vi "sub_SDR_mod.vi"(10 "Array":i16[](array[numeric]), 11 "Modulation Type":enum16{"BPSK", "4-QAM", "16-QAM", "64-QAM"}(ring)) -> (2 "Array out":cdb[](array[numeric]))   [LabVIEW 2012]
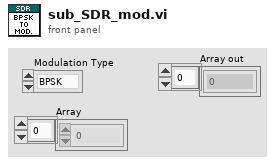
[diagram p1: front panel]
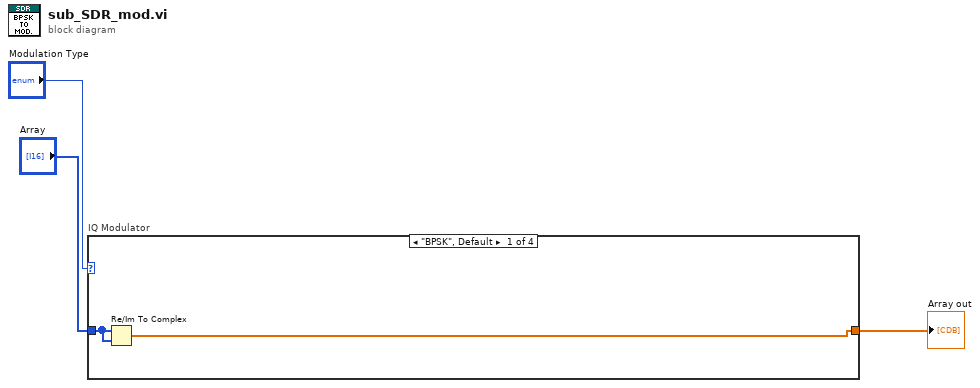
[diagram p0: block diagram]
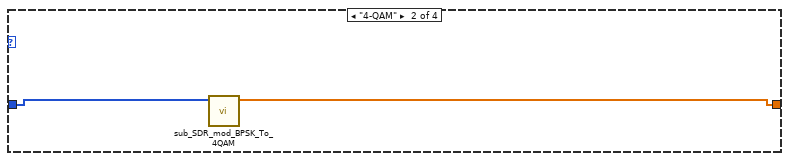
[diagram p2: hidden frame]
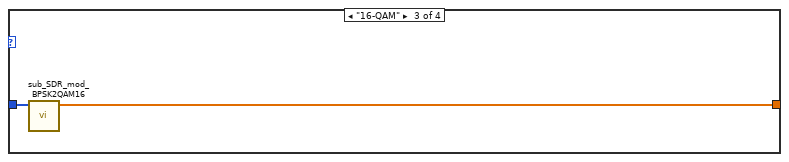
[diagram p3: hidden frame]
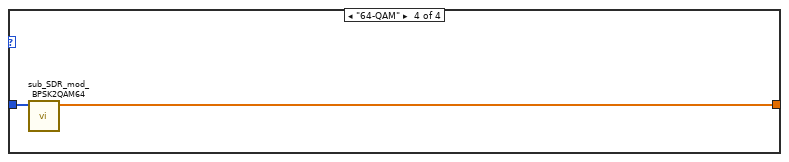
[diagram p4: hidden frame]
diagram:
  n1 = case "IQ Modulator" shown="\"BPSK\", Default" "Modulation Type" {
    tunnel: "Array" -> [w5 w6 w9 w10]
    tunnel: [w4 w7 w8 w11] -> w2
    frame "BPSK", Default {
      # "BPSK Modulator: Convert each input byte array into bolean arrays, sets phase and convert into complex"
      n2 = Re/Im To Complex(1:w5, 2:w5) -> (0:w4:cdb[])
    }
    frame "4-QAM" {
      # "4-QAM Modulator: Convert each byte in 4 integers which are maped in the defined symbols"
      n3 = call "sub_SDR_mod_BPSK_To_4QAM.vi"("Array in"=w6) -> ("Array out"=w7:cdb[])  [unwired: 10 in]
    }
    frame "16-QAM" {
      # "16-QAM Modulator: Convert each byte in 4 integers which are maped in a 4-MSK and build the phase and quadrature after"
      n4 = call "sub_SDR_mod_BPSK2QAM16.vi"("Array in"=w9) -> ("Array out"=w8:cdb[])  [unwired: 10 in]
    }
    frame "64-QAM" {
      n5 = call "sub_SDR_mod_BPSK2QAM64.vi"("Array in"=w10) -> ("Array out"=w11:cdb[])  [unwired: 10 in]
    }
  }
  "Array out" <- w2
